vi "test Value in Range (DBL).vi"(8 "error in":errorcluster, 11 "TestCase in":refnum<class "SharedUtilities.lvclass">=refnum) -> (0 "error out":errorcluster, 3 "TestCase out":refnum<class "SharedUtilities.lvclass">)   [LabVIEW 2024, in "SharedUtilities.lvclass"]
uses:
  SharedUtilities.lvclass
  decddfe9-825c-4f16-8e4d-db8670800fd4.vi
  db613d81-27a1-4f3b-8c0d-6bfb8939e49e.vi
  28217ea1-5eb1-44ab-a223-d0483fdad999.vi
  2f9decbb-61dc-432b-af07-d26697e12cc8.vi
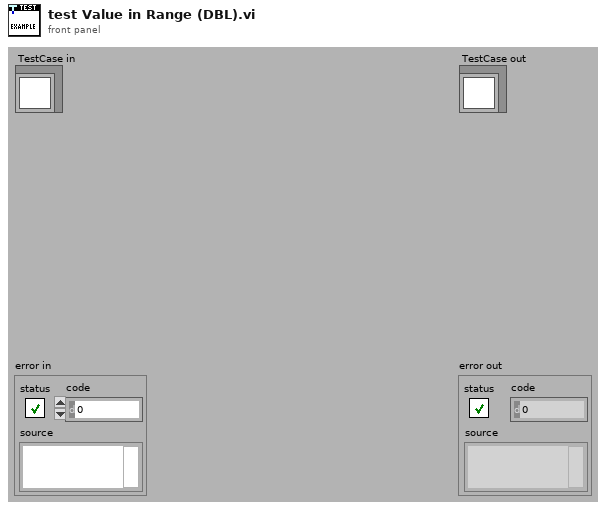
[diagram p1: front panel]
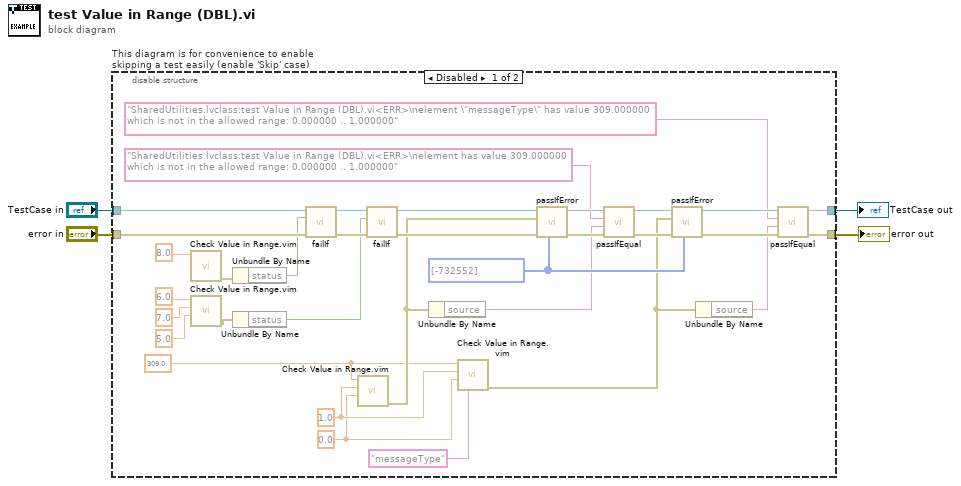
[diagram p0: block diagram]
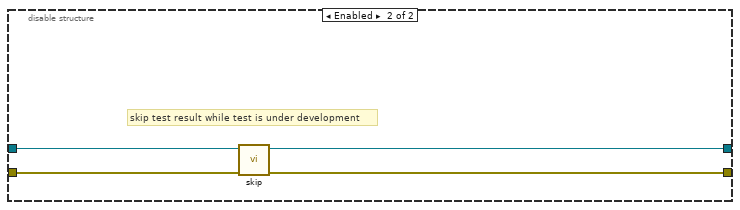
[diagram p2: hidden frame]
diagram:
  n1 = disable-structure "This diagram is for convenience to enable skipping a test easily (enable 'Skip' case)" shown="Disabled" {
    disable-tunnel: "TestCase in" -> [w33 w41]
    disable-tunnel: [w21 w39] -> w1
    disable-tunnel: [w22 w40] -> w3
    disable-tunnel: "error in" -> [w32 w38]
    frame Disabled {
      w29 = i32[] [-732552] ("passing error codes (default = any error code)")
      w5 = 0.0
      w6 = 1.0
      w7 = 309.0
      n2 = call "Check Value in Range.vim"("value"=8.0) -> ("error out"=w15:errorcluster)  [unwired: 10 in]
      n3 = call "Check Value in Range.vim"("lower limit (0)"=5.0, "upper limit (31)"=7.0, "value"=6.0) -> ("error out"=w14:errorcluster)  [unwired: 8 in]
      n4 = Unbundle By Name(w15) -> ("status"=w31:bool)
      n5 = Unbundle By Name(w14) -> ("status"=w30:bool)
      n6 = call-dynamic "failIf.vi"("error in (no error)"=w32, "fail"=w31, "TestCase in"=w33) -> ("error out"=w35:errorcluster, "TestCase out"=w34:refnum<class "SharedUtilities.lvclass">)  [unwired: 7 in]
      n7 = call "Check Value in Range.vim"("lower limit (0)"=w5, "upper limit (31)"=w6, "value"=w7) -> ("error out"=w8:errorcluster)  [unwired: 8 in]
      n8 = call-dynamic "failIf.vi"("error in (no error)"=w35, "fail"=w30, "TestCase in"=w34) -> ("error out"=w37:errorcluster, "TestCase out"=w36:refnum<class "SharedUtilities.lvclass">)  [unwired: 7 in]
      n9 = Unbundle By Name(w8) -> ("source"=w20:string)
      n10 = call "Check Value in Range.vim"("element name"="messageType", "lower limit (0)"=w5, "upper limit (31)"=w6, "value"=w7) -> ("error out"=w10:errorcluster)  [unwired: 7 in]
      n11 = call-dynamic "passIfError.vi"("passing error codes (default = any error code)"=w29, "error in (no error)"=w37, "error"=w8, "TestCase in"=w36) -> ("error out"=w28:errorcluster, "TestCase out"=w27:refnum<class "SharedUtilities.lvclass">)  [unwired: 6 in]
      n12 = call-dynamic "passIfEqual.vi"("error in (no error)"=w28, "y"=w20, "x"="SharedUtilities.lvclass:test Value in Range (DBL).vi<ERR>\nelement has value 309.000000 which is not in the allowed range: 0.000000 .. 1.000000" ("Display"), "TestCase in"=w27) -> ("error out"=w25:errorcluster, "TestCase out"=w26:refnum<class "SharedUtilities.lvclass">)  [unwired: 6 in]
      n13 = call-dynamic "passIfError.vi"("passing error codes (default = any error code)"=w29, "error in (no error)"=w25, "error"=w10, "TestCase in"=w26) -> ("error out"=w23:errorcluster, "TestCase out"=w24:refnum<class "SharedUtilities.lvclass">)  [unwired: 6 in]
      n14 = Unbundle By Name(w10) -> ("source"=w19:string)
      n15 = call-dynamic "passIfEqual.vi"("error in (no error)"=w23, "y"=w19, "x"="SharedUtilities.lvclass:test Value in Range (DBL).vi<ERR>\nelement \"messageType\" has value 309.000000 which is not in the allowed range: 0.000000 .. 1.000000" ("Display"), "TestCase in"=w24) -> ("error out"=w22:errorcluster, "TestCase out"=w21:refnum<class "SharedUtilities.lvclass">)  [unwired: 6 in]
    }
    frame Enabled {
      # "skip test result while test is under development"
      n16 = call <vilib>:"skip.vi"("error in (no error)"=w38, "TestCase in"=w41) -> ("error out"=w40:errorcluster, "TestCase out"=w39:refnum<class "SharedUtilities.lvclass">)  [unwired: 8 in]
    }
  }
  "error out" <- w3
  "TestCase out" <- w1
